vi "绘制方块.vi"(9 "簇":cluster{"行":dbl, "列":dbl}, 10 "ID":i32, 11 "picture":picture caption="图片") -> (3 "new picture":picture caption="新图片")   [LabVIEW 2012]
uses:
  <vilib>/picture/picture.llb/Draw True-Color Pixmap.vi
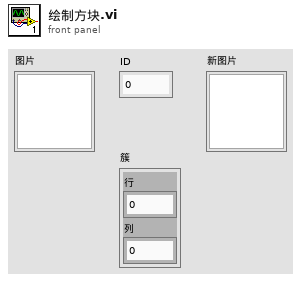
[diagram p1: front panel]
types:
  T1 = cluster{"数组":i32[][][], "colors":u32[], "mask":u8[]}
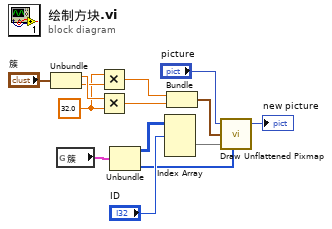
[diagram p0: block diagram]
diagram:
  w11 = 32.0 ("y")
  n1 = Unbundle("簇") -> ("行"=w13:dbl, "列"=w12:dbl)
  n2 = global read "全局变量.vi" "簇"() -> (w1:T1)
  n3 = Multiply(x=w11, y=w12) -> (x*y=w4:dbl)
  n4 = Multiply(x=w13, y=w11) -> (x*y=w5:dbl)
  n5 = Unbundle(w1) -> ("数组"=w7:i32[][][], "mask"=w6:u8[])  [unwired: 1 out]
  n6 = Index Array(array=w7, index (dim 0)="ID") -> (element=w8:i32[][])  [unwired: 2 in]
  n7 = Bundle(w4, w5) -> (w10:cluster{dbl, dbl})  [unwired: 1 in]
  n8 = call-poly <vilib>:"Draw Unflattened Pixmap.vi"("picture"="picture", "top left point(0, 0)"=w10, "data (RGB format)"=w8, "mask"=w6) -> ("new picture"=→"new picture":picture)  [unwired: 5 in]
